vi "Read Boolean.vi"(8 "error in (no error)":errorcluster, 11 "ExampleClass2 in":refnum<class "ExampleClass2.lvclass">) -> (0 "error out":errorcluster, 2 "Numeric":dbl, 3 "ExampleClass2 out":refnum<class "ExampleClass2.lvclass">)   [LabVIEW 2014, in "ExampleClass2.lvclass"]
uses:
  ExampleClass2.lvclass
  ExampleClass2.lvclass/ExampleClass2.ctl
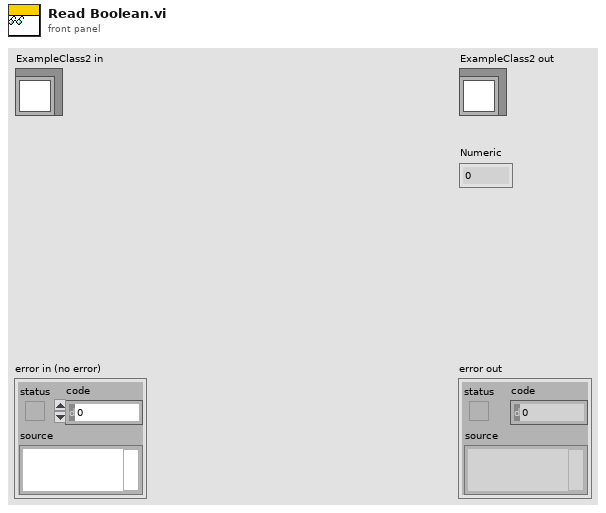
[diagram p1: front panel]
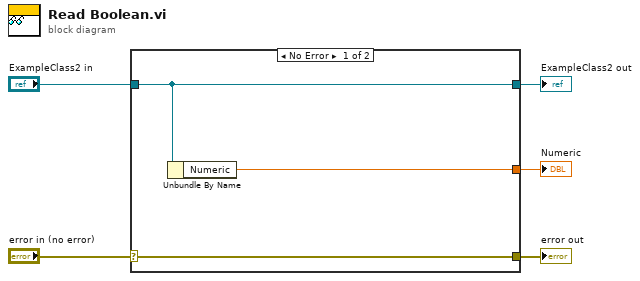
[diagram p0: block diagram]
diagram:
  n1 = case shown="No Error" "error in (no error)" {
    selector: "error in (no error)" -> [w8 w9]
    tunnel: [w8 w9] -> w4
    tunnel: [w7 w10] -> w2
    tunnel: "ExampleClass2 in" -> [w7 w10]
    tunnel: [w6 _] -> w1
    frame No Error {
      n2 = Unbundle By Name(w7) -> ("Numeric"=w6:dbl)
    }
    frame Error {
    }
  }
  "error out" <- w4
  "ExampleClass2 out" <- w2
  "Numeric" <- w1
